vi "BuilFFT_cluster.vi"(6 "Enum":enum16{"by dF", "by dX"}(ring), 8 "input Y":dbl=0.1 format="%#_13g", 9 "input X":dbl=0.1 format="%#_13g", 10 "Ny":i32=1024, 11 "Nx":i32=1024) -> (3 "fft cluster":T1)   [LabVIEW 2018, in "myFFT.lvlib"]
uses:
  myFFT.lvlib
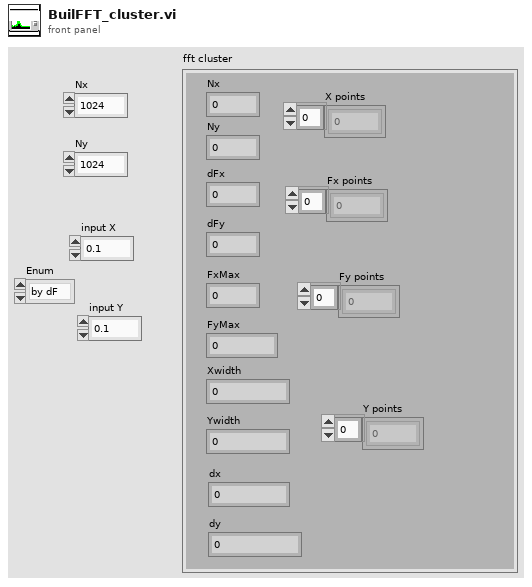
[diagram p1: front panel]
types:
  T1 = cluster{"dFx":dbl, "dFy":dbl, "Nx":i32, "Ny":i32, "FxMax":dbl, "FyMax":dbl, "Xwidth":dbl, "Ywidth":dbl, "dx":dbl, "dy":dbl, "Fx points":dbl[], "X points":dbl[], "Y points":dbl[], "Fy points":dbl[]}
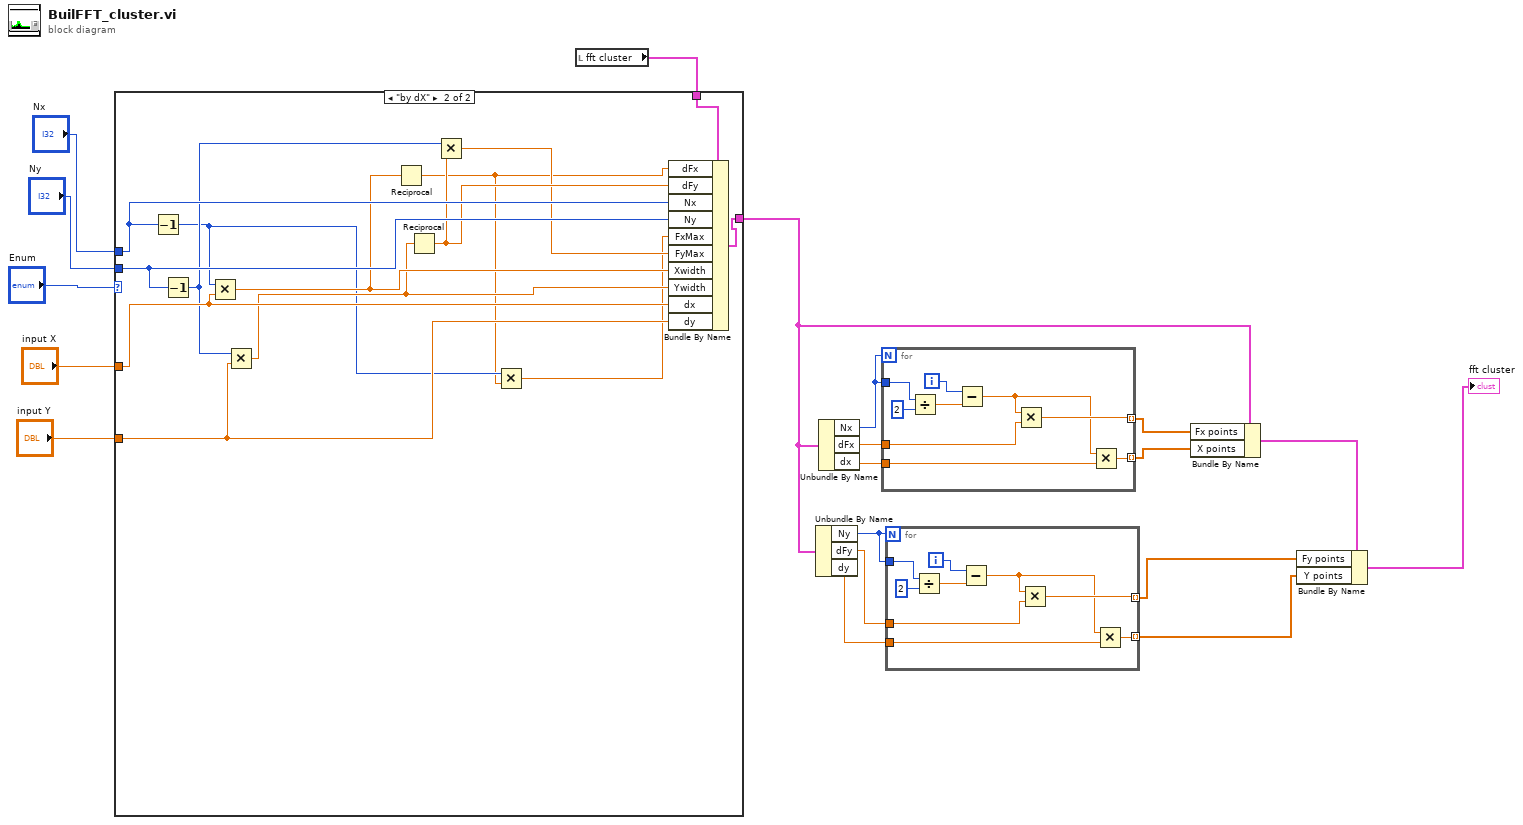
[diagram p0: block diagram]
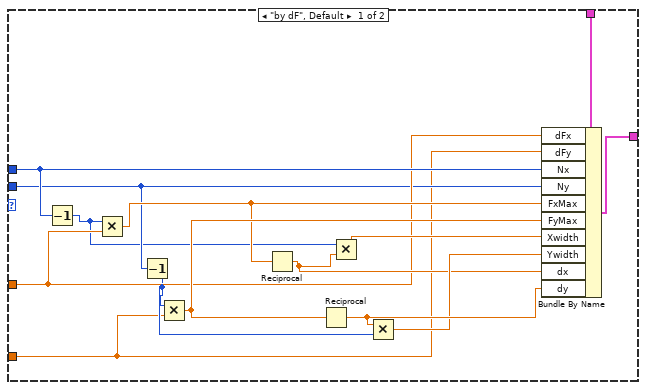
[diagram p2: hidden frame]
diagram:
  n1 = local read "fft cluster"() -> (w2:T1)
  n2 = case shown="\"by dX\"" "Enum" {
    tunnel: [w33 w46] -> w9
    tunnel: "input X" -> [w25 w43]
    tunnel: "input Y" -> [w21 w42]
    tunnel: "Nx" -> [w26 w45]
    tunnel: "Ny" -> [w24 w44]
    tunnel: w2 -> [w20 w47]
    frame "by dF", Default {
      n3 = Decrement(x=w26) -> (x-1=w23:i32)
      n4 = Multiply(x=w23, y=w25) -> (x*y=w31:dbl)
      n5 = Decrement(x=w24) -> (x-1=w22:i32)
      n6 = Multiply(x=w22, y=w21) -> (x*y=w32:dbl)
      n7 = Reciprocal(x=w31) -> (1/x=w27:dbl)
      n8 = Reciprocal(x=w32) -> (1/x=w30:dbl)
      n9 = Multiply(x=w23, y=w27) -> (x*y=w28:dbl)
      n10 = Multiply(x=w30, y=w22) -> (x*y=w29:dbl)
      n11 = Bundle By Name(cluster=w20, "dFx"=w25, "dFy"=w21, "Nx"=w26, "Ny"=w24, "FxMax"=w31, "FyMax"=w32, "Xwidth"=w28, "Ywidth"=w29, "dx"=w27, "dy"=w30) -> (w33:T1)
    }
    frame "by dX" {
      n12 = Decrement(x=w45) -> (x-1=w35:i32)
      n13 = Decrement(x=w44) -> (x-1=w38:i32)
      n14 = Multiply(x=w35, y=w43) -> (x*y=w41:dbl)
      n15 = Multiply(x=w38, y=w42) -> (x*y=w40:dbl)
      n16 = Reciprocal(x=w41) -> (1/x=w34:dbl)
      n17 = Reciprocal(x=w40) -> (1/x=w39:dbl)
      n18 = Multiply(x=w38, y=w39) -> (x*y=w37:dbl)
      n19 = Multiply(x=w35, y=w34) -> (x*y=w36:dbl)
      n20 = Bundle By Name(cluster=w47, "dFx"=w34, "dFy"=w39, "Nx"=w45, "Ny"=w44, "FxMax"=w36, "FyMax"=w37, "Xwidth"=w41, "Ywidth"=w40, "dx"=w43, "dy"=w42) -> (w46:T1)
    }
  }
  n21 = Unbundle By Name(w9) -> ("Ny"=w6:i32, "dFy"=w8:dbl, "dy"=w7:dbl)
  n22 = Unbundle By Name(w9) -> ("Nx"=w14:i32, "dFx"=w13:dbl, "dx"=w12:dbl)
  n23 = for {
    N: w14 -> [_]
    tunnel: w14 -> [w54]
    tunnel: w13 -> [w52]
    tunnel: [w51] -> w11 mode=indexing
    tunnel: w12 -> [w49]
    tunnel: [w48] -> w10 mode=indexing
    i -> [w56]
    n24 = Divide(x=w54, y=2) -> (x/y=w55:dbl)
    n25 = Subtract(x=w56, y=w55) -> (x-y=w50:dbl)
    n26 = Multiply(x=w50, y=w52) -> (x*y=w51:dbl)
    n27 = Multiply(x=w50, y=w49) -> (x*y=w48:dbl)
  }
  n28 = for {
    N: w6 -> [_]
    tunnel: w6 -> [w63]
    tunnel: w8 -> [w61]
    tunnel: [w60] -> w1 mode=indexing
    tunnel: w7 -> [w58]
    tunnel: [w57] -> w5 mode=indexing
    i -> [w65]
    n29 = Divide(x=w63, y=2) -> (x/y=w64:dbl)
    n30 = Subtract(x=w65, y=w64) -> (x-y=w59:dbl)
    n31 = Multiply(x=w59, y=w61) -> (x*y=w60:dbl)
    n32 = Multiply(x=w59, y=w58) -> (x*y=w57:dbl)
  }
  n33 = Bundle By Name(cluster=w9, "Fx points"=w11, "X points"=w10) -> (w4:T1)
  n34 = Bundle By Name(cluster=w4, "Fy points"=w1, "Y points"=w5) -> (→"fft cluster":T1)
